vi "PKYK_RFID_BUILDER.vi"(5 "TS Parameter":T1={"ProfitCenterCode"="", "LineCode"="", "WorkOrderNumber"="", "Model"="", "Model_with_Prefix"="", "VendorCode"="", "SetParameterDateCode"="", "PokaYoke"=0, "Target"=1, "Live_DateCode"="", "CustomerPartNumber"="", "Hand"="", "sBarcode"=FALSE, "FCA"=0, "Ent_Stamp"=timestamp(0 s since 1904-01-01), "STS_CD"=0.0} {"FCA" format="%01d"; "Target" min=1 max=100000; "PokaYoke" min=0 max=1}, 7 "Pokeyoke?":bool[](array[boolean]), 8 "error in (no error)":errorcluster, 11 "MS SQL Connection In":T2) -> (0 "error out":errorcluster, 3 "MS SQL Connection Out":T2)   [LabVIEW 2020]
uses:
  <vilib>/addons/database/Connection.llb/Conn ObjectReference.ctl
  Controls/TS_Parameter.ctl
  MS SQL/MS_Global.vi
  <vilib>/addons/database/NI_Database_API.lvlib
panel:
  out "data":variant[][](array[variant])
  out "Array 3":bool[][](array[boolean])
  out "Array 2":timestamp[][](array[timestamp])
  out "Array":string[][](array[string])
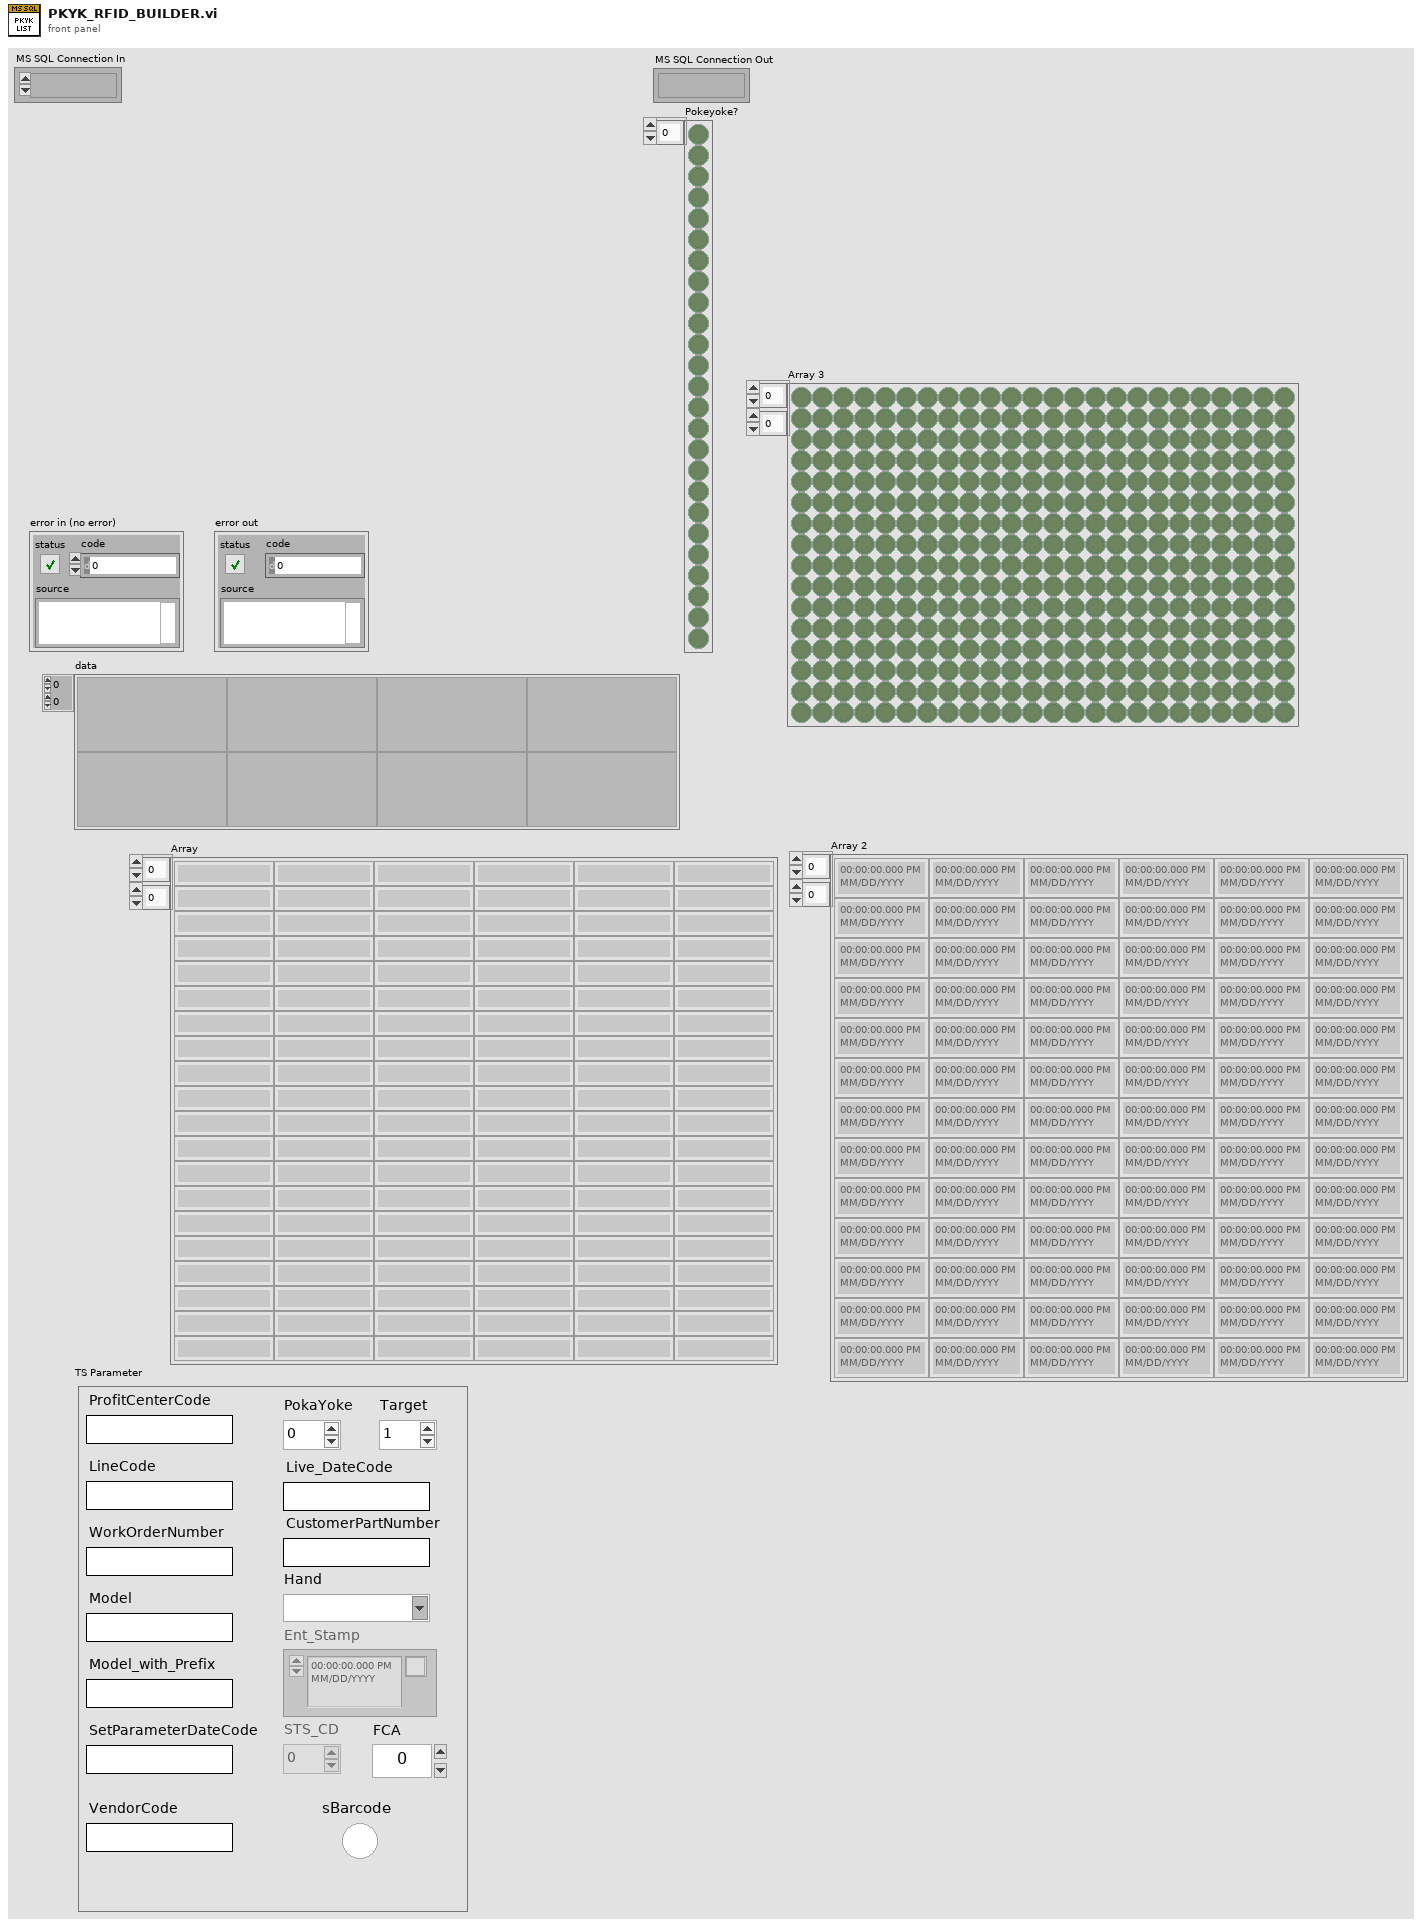
[diagram p1: front panel]
types:
  T1 = typedef "TS_Parameter.ctl" = cluster{"ProfitCenterCode":string, "LineCode":string, "WorkOrderNumber":string, "Model":string, "Model_with_Prefix":string, "VendorCode":string, "SetParameterDateCode":string, "PokaYoke":i32, "Target":i32, "Live_DateCode":string, "CustomerPartNumber":string, "Hand":string, "sBarcode":bool, "FCA":i32, "Ent_Stamp":timestamp, "STS_CD":dbl}
  T2 = typedef "NI_Database_API.lvlib/Conn ObjectReference.ctl" = refnum<k1>
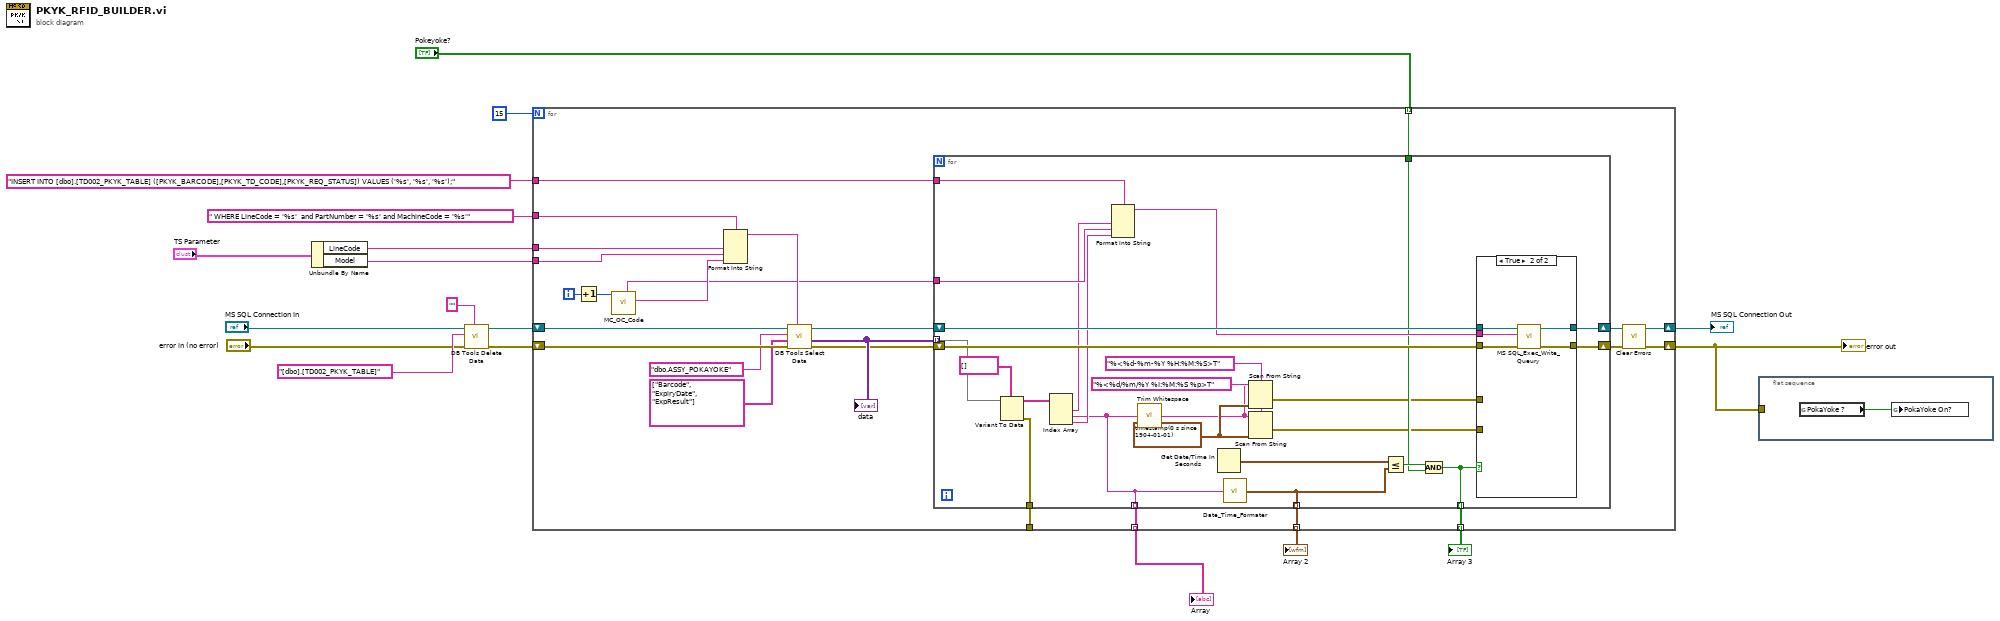
[diagram p0: block diagram]
diagram:
  n1 = Unbundle By Name("TS Parameter") -> ("LineCode"=w2:string, "Model"=w1:string)
  n2 = call <vilib>:"DB Tools Delete Data.vi"("condition"="", "error in (no error)"="error in (no error)", "table"="[dbo].[TD002_PKYK_TABLE]", "connection reference"="MS SQL Connection In") -> ("error out"=w13:errorcluster, "connection reference out"=w15:T2)  [unwired: 6 in]
  n3 = for {
    N: 15 -> [_]
    tunnel: " WHERE LineCode = '%s'  and PartNumber = '%s' and MachineCode = '%s'" -> [w42]
    shift-right: [w34] -> w12
    shift-left: w15 -> [w41]
    shift-right: [w29] -> w4
    shift-left: w13 -> [w40]
    tunnel: "INSERT INTO [dbo].[TD002_PKYK_TABLE] ([PKYK_BARCODE],[PKYK_TD_CODE],[PKYK_REQ_STATUS]) VALUES ('%s', '%s', '%s');" ("Query") -> [w28]
    tunnel: "Pokeyoke?" -> [w27] mode=indexing
    tunnel: [w26] -> _
    tunnel: [w25] -> w8 mode=indexing
    tunnel: [w24] -> w7 mode=indexing
    tunnel: [w23] -> w6 mode=indexing
    tunnel: w2 -> [w20]
    tunnel: w1 -> [w19]
    i -> [w31]
    n4 = Increment(x=w31) -> (x+1=w30:i32)
    n5 = call "MC_OC_Code.vi"("index"=w30) -> ("Machine Code"=w22:string, "Machine No."=w21:string)  [unwired: 4 in, 5 out]
    n6 = Format Into String(format string=w42, w20, w19, w22) -> (resulting string=w39:string)  [unwired: 2 in, 1 out]
    n7 = call <vilib>:"DB Tools Select Data.vi"("condition"=w39, "error in (no error)"=w40, "columns"=string[] ["Barcode", "ExpiryDate", "ExpResult"], "table"="dbo.ASSY_POKAYOKE", "connection reference"=w41) -> ("error out"=w33:errorcluster, "data"=w37:variant[][], "connection reference out"=w35:T2)  [unwired: 1 in]
    "data" <- w37
    n8 = for {
      tunnel: w37 -> [w55] mode=indexing
      tunnel: w21 -> [w58]
      tunnel: w28 -> [w56]
      shift-right: [w63] -> w34
      shift-left: w35 -> [w64]
      shift-right: [w61] -> w32
      shift-left: w33 -> [w62]
      tunnel: w27 -> [w54]
      tunnel: [w52] -> w26
      tunnel: [w45] -> w25 mode=indexing
      tunnel: [w44] -> w24 mode=indexing
      tunnel: [w43] -> w23 mode=indexing
      w49 = timestamp(0 s since 1904-01-01) ("time stamp")
      n9 = Variant To Data(type=string[] [], Variant=w55) -> (data=w53:string[], error out=w52:errorcluster)  [unwired: 1 in]
      n10 = Index Array(array=w53) -> (element #1=w51:string, element #2=w45:string, element #3=w57:string)  [unwired: 3 in]
      n11 = Format Into String(format string=w56, w51, w58, w57) -> (resulting string=w59:string)  [unwired: 2 in, 1 out]
      n12 = call <vilib>:"Trim Whitespace.vi"("string"=w45) -> ("trimmed string"=w46:string)  [unwired: 1 in]
      n13 = Get Date/Time In Seconds() -> (seconds since 1Jan1904=w65:timestamp)
      n14 = call "Date_Time_Formater.vi"("Date In"=w45) -> ("Date Out"=w44:timestamp)
      n15 = Scan From String(format string="%<%d-%m-%Y %H:%M:%S>T" ("time format string (%c)"), input string=w46, default 1=w49) -> (error out=w48:errorcluster)  [unwired: 3 in, 2 out]
      n16 = Scan From String(format string="%<%d/%m/%Y %I:%M:%S %p>T" ("time format string (%c)"), input string=w46, default 1=w49) -> (error out=w47:errorcluster)  [unwired: 3 in, 2 out]
      n17 = Less Or Equal?(x=w65, y=w44) -> (x <= y?=w60:bool)
      n18 = Compound Arithmetic op=AND(w60, w54) -> (w43:bool)
      n19 = case shown="True" w43 {
        tunnel: w64 -> [w69 w74]
        tunnel: [w69 w73] -> w63
        tunnel: w62 -> [w68 w72]
        tunnel: [w68 w71] -> w61
        tunnel: w59 -> [_ w70]
        tunnel: w47 -> [_ _]
        tunnel: w48 -> [_ _]
        frame False {
        }
        frame True {
          n20 = call "MS SQL_Exec_Write_Queury.vi"("error in (no error)"=w72, "Query"=w70, "Refnum in"=w74) -> ("error out"=w71:errorcluster, "Refnum out"=w73:T2)  [unwired: 7 in]
        }
      }
    }
    n21 = call <vilib>:"Clear Errors.vi"("error in (no error)"=w32) -> ("error out"=w29:errorcluster)  [unwired: 5 in, 1 out]
  }
  "error out" <- w4
  "MS SQL Connection Out" <- w12
  "Array" <- w8
  "Array 2" <- w7
  "Array 3" <- w6
  n22 = flat-sequence {
    tunnel: w4 -> [_]
    frame #0 {
      n23 = global read "MS_Global.vi" "PokaYoke ?"() -> (w75:bool)
      n24 = global write "MS_Global.vi" "PokaYoke On?"(w75) -> ()
    }
  }
